vi "Unpack Notification Msg.vi"(11 "Notification Msg":refnum<class "Notification Msg.lvclass">) -> (1 "Publication Time":timestamp, 2 "Value":variant, 3 "Datum Name":string)   [LabVIEW 2017, in "Transport.lvlib" / "Notification Msg.lvclass"]
doc: "<License>\nCopyright © 2017 Composed Systems, LLC | All rights reserved\nwww.composed.io\n\nAuthor: Ethan Stern <ethan.stern@composed.io>\n\nThis software is provided \"AS IS\" WITHOUT WARRANTIES, either express or implied, AND IS FOR EDUCATIONAL PURPOSES ONLY.\n</License>"
uses:
  Notification Msg.lvclass
  gpm_packages/@cs/transport/Source/Concrete/ActorMessageTransport/Notification Msg/Notification Msg.lvclass
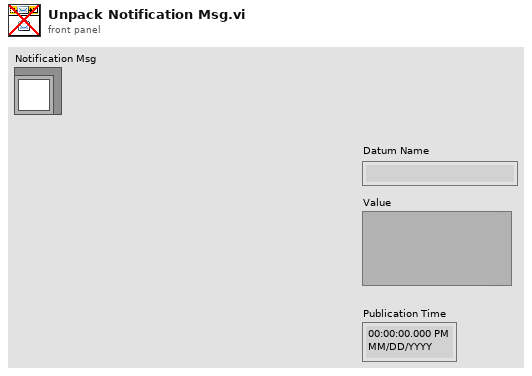
[diagram p1: front panel]
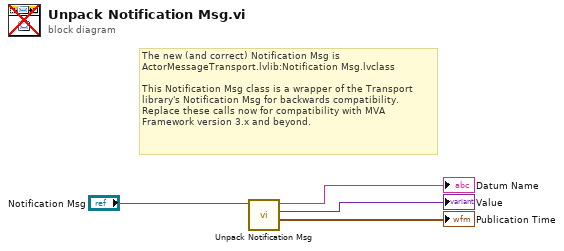
[diagram p0: block diagram]
diagram:
  # "The new (and correct) Notification Msg is\nActorMessageTransport.lvlib:Notification Msg.lvclass\n\nThis Notification Msg class is a wrapper of the Transport\nlibrary's Notification Msg for backwards compatibility.\nReplace these calls now for compatibility with MVA\nFramework version 3.x and beyond."
  n1 = call-parent "Unpack Notification Msg.vi"("Notification Msg"="Notification Msg") -> ("Publication Time"=→"Publication Time":timestamp, "Value"=→"Value":variant, "Datum Name"=→"Datum Name":string)  [unwired: 8 in]
